vi "DG535.get C mode.vi"(0 "i ref in":refnum<vi>, 11 "error in (no error)":errorcluster) -> (4 "i ref out":refnum<vi>, 8 "mode":i32(ring) items=["TTL", "NIM", "ECL", "VAR"], 15 "error out":errorcluster)   [LabVIEW 2014, in "DG535.lvlib"]
uses:
  DG535.lvlib
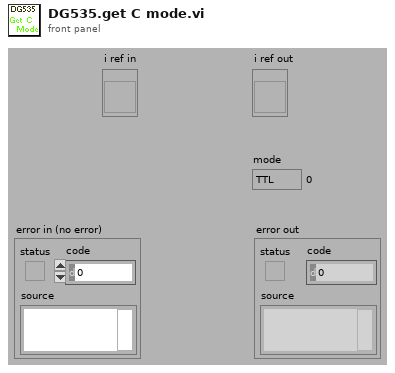
[diagram p1: front panel]
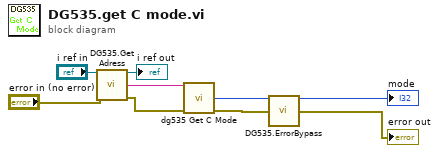
[diagram p0: block diagram]
diagram:
  n1 = call "DG535.Get Adress.vi"("i ref in"="i ref in", "error in (no error)"="error in (no error)") -> ("i ref out"=→"i ref out":refnum<vi>, "address"=w5:string, "error out"=w4:errorcluster)  [unwired: 10 in, 1 out]
  n2 = call "dg535 Get C Mode.vi"("address string"=w5, "error in"=w4) -> ("mode"=→"mode":i32, "error out"=w3:errorcluster)  [unwired: 12 in]
  n3 = call "DG535.ErrorBypass.vi"("error in (no error)"=w3) -> ("error out"=→"error out":errorcluster)  [unwired: 14 in]
